vi "message_postie.vi"(0 "HGF_Reference":refnum<class "HGF_Reference.lvclass">, 3 "String":string, 5 "error IO":errorcluster, 6 "timeout in ms (-1)":i32) -> (16 "TEST_addressee":string, 17 "TEST_receiver":T1(ring), 19 "error out":errorcluster)   [LabVIEW 2009, in "MoAgSy.lvlib" / "MoAgSy_Host.lvclass"]
doc: "NOT YET FINISHED\nSend reply if receiver is unknown,\nif receiver is host, this VI adds message to hosts internal queue\n\nF.Berck@gsi.de\nGSI Darmstadt 2009"
uses:
  MoAgSy_Host.lvclass
  HGF_BaseClasses/HGF_Reference/HGF_Reference.lvclass
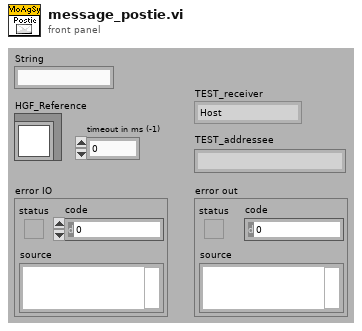
[diagram p1: front panel]
types:
  T1 = enum16{"Host", "running agent", "past Agent", "unknown"}
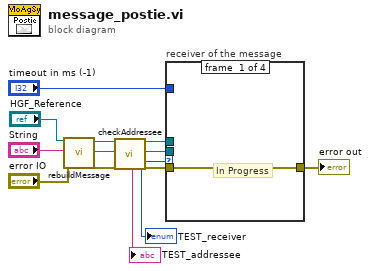
[diagram p0: block diagram]
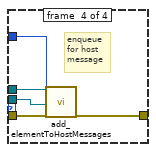
[diagram p4: hidden frame]
diagram:
  n1 = call "rebuildMessage.vi"("Host_Reference"="HGF_Reference", "Object Data"="String", "error in (no error)"="error IO") -> ("dup HGF_Reference"=w3:refnum<class "HGF_Reference.lvclass">, "MoAgSy_Message"=w4:refnum<class "MoAgSy_Message.lvclass">, "error out"=w5:errorcluster)  [unwired: 2 in, 12 out]
  n2 = call "checkAddressee.vi"("Host_Reference"=w3, "MoAgSy_Message"=w4, "error in (no error)"=w5) -> ("addressee"=→"TEST_addressee":string, "dup HGF_Reference"=w10:refnum<class "HGF_Reference.lvclass">, "dup MoAgSy_Message"=w11:refnum<class "MoAgSy_Message.lvclass">, "receiver"=w7:T1, "error out"=w9:errorcluster)  [unwired: 12 out]
  "TEST_receiver" <- w7
  n3 = case "receiver of the message" shown="\"Host\"" w7 {
    tunnel: [w14 w15 w16 w18] -> w8
    tunnel: w9 -> [w14 w15 w16 w21]
    tunnel: w10 -> [_ _ _ w20]
    tunnel: w11 -> [_ _ _ w19]
    tunnel: "timeout in ms (-1)" -> [_ _ _ w17]
    frame #0 {
      # "In Progress"
    }
    frame #1 {
      # "In Progress"
    }
    frame #2 {
      # "In Progress"
    }
    frame #3 {
      # "enqueue\nfor host\nmessage"
      n4 = call "add_elementToHostMessages.vi"("Host_Reference"=w20, "timeout in ms (-1)"=w17, "MoAgSy_Message"=w19, "error in (no error)"=w21) -> ("error out"=w18:errorcluster)  [unwired: 15 out]
    }
  }
  "error out" <- w8
